vi "Auto_NFC_TCPIP.vi"(9 "error in":errorcluster, 10 "connection ID in":refnum<k5>) -> (0 "error out":errorcluster, 1 "Read Data":string, 2 "UID":string, 3 "connection ID out":refnum<k5>, 4 "x .and. y?":bool)   [LabVIEW 2017]
panel:
  in  "Read":string="RD_01_00000_0015"
  out "Response":string
  out "Init 2":string
  out "Init":string
  in  "Init":string="CU_00_00_00_00_00_AS"
  in  "configure channel":string="CI_01_11_0000_004_064_01_01_00"
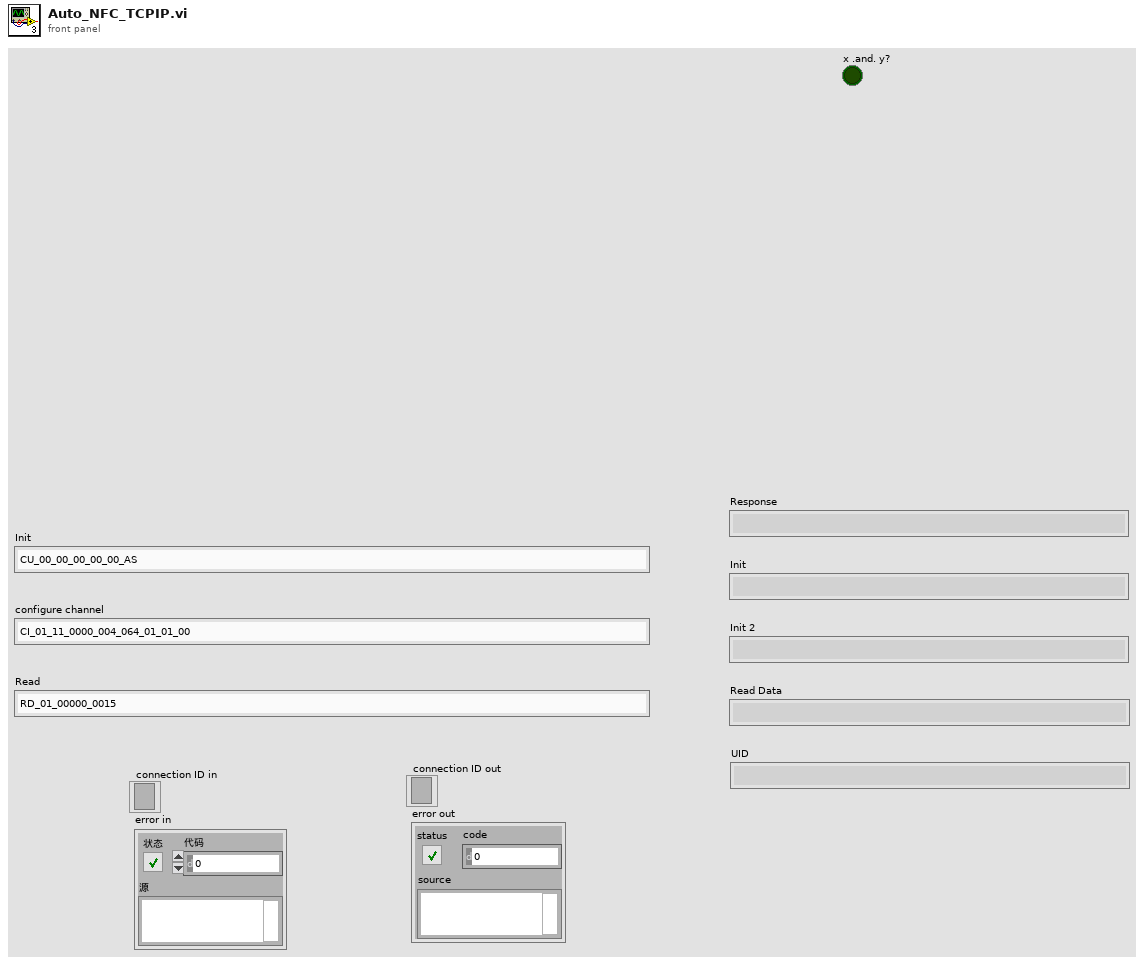
[diagram p1: front panel]
types:
  T1 = cluster{"Check UID":string, "NFC tag memory blocks 00 – 31":string, "NFC tag memory blocks 32 – 63":string, "Read Fixture ID":string, "Read UID":string, "Read Memory block":string, "Read Block size":string, "Read user data and verify bocks 00 - 31":string, "Read user data and verify bocks 32 - 63":string, "Memory secured by disabling the write access":string, "Verify the memory is secured":string, "Read user data and verify the memory (256 bytes) ":string}
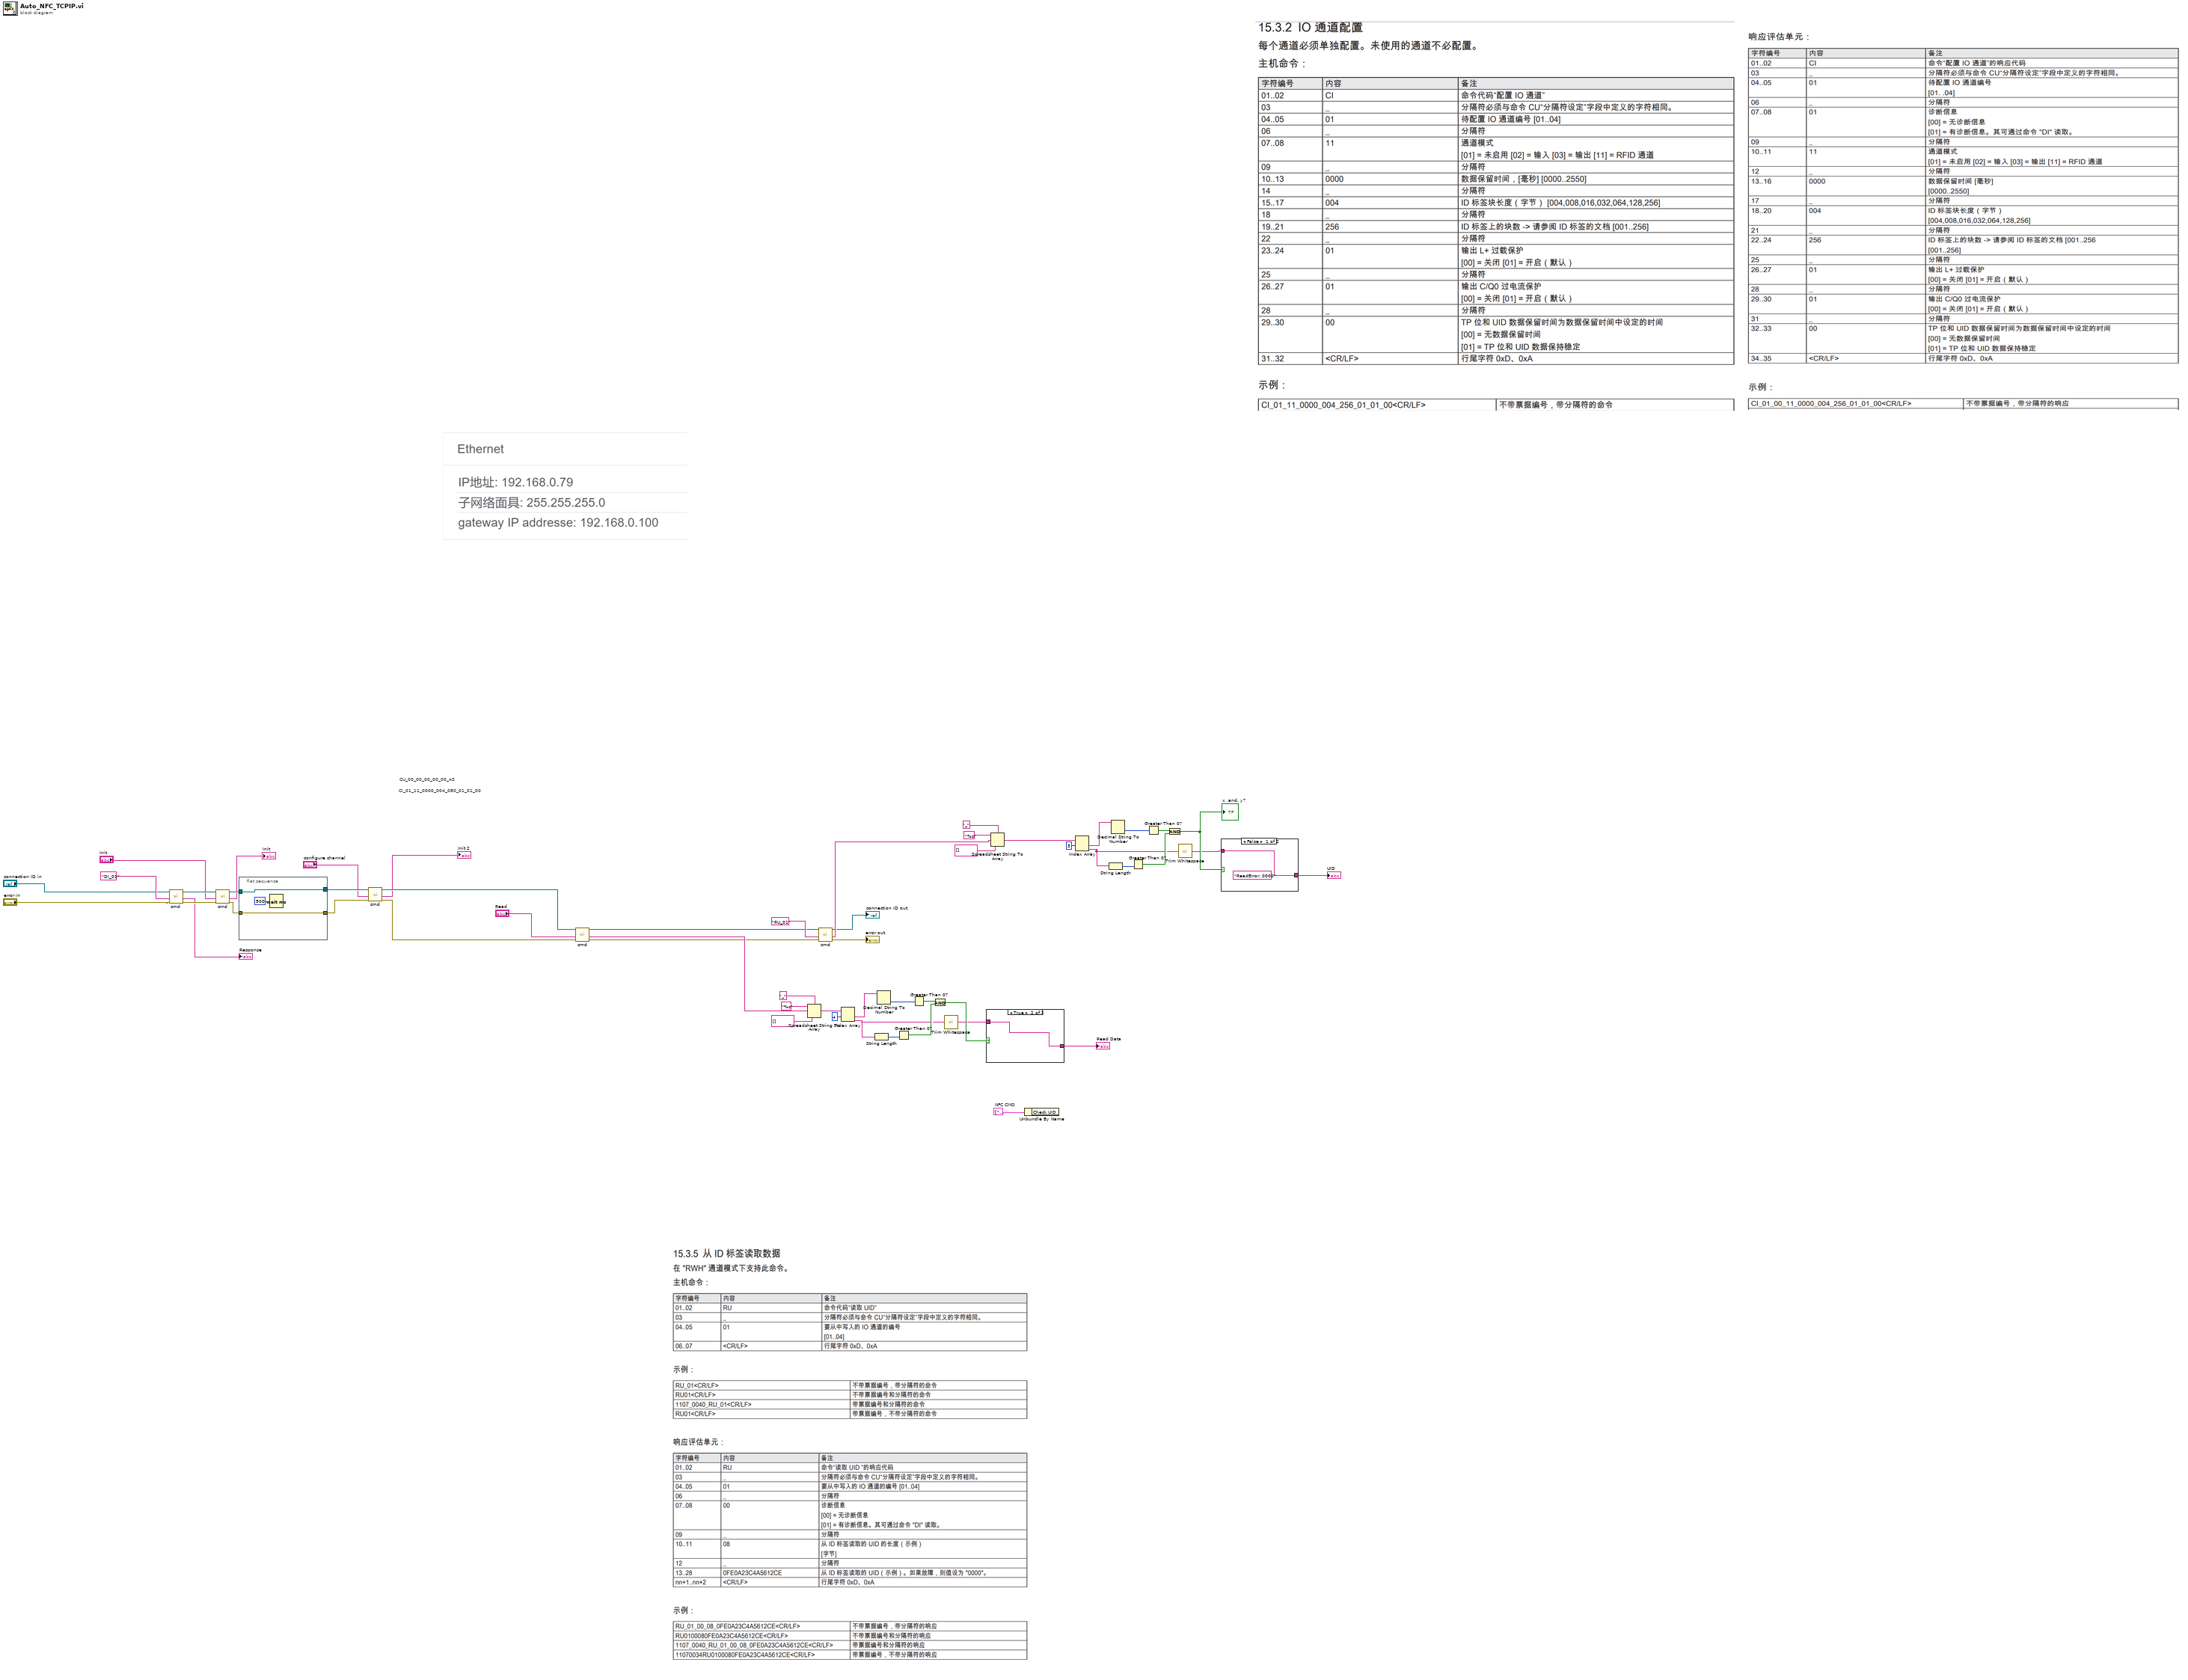
[diagram p0: block diagram]
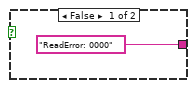
[diagram p3: hidden frame]
diagram:
  w47 = T1 {"Check UID"="ACCESSORY_TAG_READ_DATA_REQ", "NFC tag memory blocks 00 – 31"="ACCESSORY_PROGRAM_CMD", "NFC tag memory blocks 32 – 63"="TBA", "Read Fixture ID"="TBA", "Read UID"="TBA", "Read Memory block"="TBA", "Read Block size"="TBA", "Read user data and verify bocks 00 - 31"="ACCESSORY_TAG_READ_DATA_REQ", "Read user data and verify bocks 32 - 63"="TBA", "Memory secured by disabling the write access"="TBA", "Verify the memory is secured"="TBA", "Read user data and verify the memory (256 bytes) "="ACCESSORY_TAG_READ_DATA_REQ"}  # NFC CMD
  # "CI_01_11_0000_004_080_01_01_00"
  # "CU_00_00_00_00_00_AS"
  n1 = call "cmd.vi"("错误输入"="error in", "Cmd"="DI_01", "连接ID"="connection ID in") -> ("错误输出"=w37:errorcluster, "Response"=→"Response":string, "连接ID输出"=w38:refnum<k5>)  [unwired: 6 in]
  n2 = call "cmd.vi"("错误输入"=w37, "Cmd"="Init", "连接ID"=w38) -> ("错误输出"=w45:errorcluster, "Response"=→"Init":string, "连接ID输出"=w46:refnum<k5>)  [unwired: 6 in]
  n3 = flat-sequence {
    tunnel: w45 -> [w55]
    tunnel: [w55] -> w43
    tunnel: w46 -> [w54]
    tunnel: [w54] -> w44
    frame #0 {
      n4 = Wait (ms)(milliseconds to wait=u32 500 ("等待时间（毫秒）")) -> ()  [unwired: 1 out]
    }
  }
  n5 = call "cmd.vi"("错误输入"=w43, "Cmd"="configure channel", "连接ID"=w44) -> ("错误输出"=w26:errorcluster, "Response"=→"Init 2":string, "连接ID输出"=w42:refnum<k5>)  [unwired: 6 in]
  n6 = call "cmd.vi"("错误输入"=w26, "Cmd"="Read", "连接ID"=w42) -> ("错误输出"=w21:errorcluster, "Response"=w41:string, "连接ID输出"=w22:refnum<k5>)  [unwired: 6 in]
  n7 = Spreadsheet String To Array(delimiter (Tab)="_" ("分隔符(Tab)"), format string="%s" ("格式字符串"), spreadsheet string=w41, array type (2D Dbl)=string[] []) -> (array=w50:string[])
  n8 = call "cmd.vi"("错误输入"=w21, "Cmd"="RU_01", "连接ID"=w22) -> ("错误输出"=→"error out":errorcluster, "Response"=w17:string, "连接ID输出"=→"connection ID out":refnum<k5>)  [unwired: 6 in]
  n9 = Index Array(array=w50, index #1=4 ("索引")) -> (element #1=w33:string, element #2=w25:string)  [unwired: 1 in]
  n10 = String Length(string=w25) -> (length=w28:i32)
  n11 = Decimal String To Number(string=w33) -> (number=w32:i32)  [unwired: 2 in, 1 out]
  n12 = Greater Than 0?(x=w28) -> (x > 0?=w30:bool)
  n13 = Greater Than 0?(x=w32) -> (x > 0?=w31:bool)
  n14 = And(x=w31, y=w30) -> (x .and. y?=w29:bool)
  n15 = call <vilib>:"Trim Whitespace.vi"("string"=w25) -> ("trimmed string"=w24:string)  [unwired: 1 in]
  n16 = case shown="True" w29 {
    tunnel: ["ReadError: 0000" ("y") w58] -> w48
    tunnel: w24 -> [_ w58]
    frame False {
    }
    frame True {
    }
  }
  "Read Data" <- w48
  n17 = Spreadsheet String To Array(delimiter (Tab)="_" ("分隔符(Tab)"), format string="%s" ("格式字符串"), spreadsheet string=w17, array type (2D Dbl)=string[] []) -> (array=w6:string[])
  n18 = Unbundle By Name(w47) -> ()  [unwired: 1 out]
  n19 = Index Array(array=w6, index #1=3 ("索引")) -> (element #1=w15:string, element #2=w9:string)  [unwired: 1 in]
  n20 = String Length(string=w9) -> (length=w10:i32)
  n21 = Decimal String To Number(string=w15) -> (number=w14:i32)  [unwired: 2 in, 1 out]
  n22 = Greater Than 0?(x=w10) -> (x > 0?=w12:bool)
  n23 = Greater Than 0?(x=w14) -> (x > 0?=w13:bool)
  n24 = And(x=w13, y=w12) -> (x .and. y?=w11:bool)
  "x .and. y?" <- w11
  n25 = call <vilib>:"Trim Whitespace.vi"("string"=w9) -> ("trimmed string"=w8:string)  [unwired: 1 in]
  n26 = case shown="False" w11 {
    tunnel: [w59 w60] -> w5
    tunnel: w8 -> [w59 w60]
    frame False {
      (unwired) "ReadError: 0000" ("y")
    }
    frame True {
    }
  }
  "UID" <- w5
